vi "Read url 1.vi"(8 "error in (no error)":errorcluster, 11 "Firebase in":refnum<class "Firebase.lvclass">) -> (0 "error out":errorcluster, 2 "url":string, 3 "Firebase out":refnum<class "Firebase.lvclass">)   [LabVIEW 2019, in "Firebase.lvclass"]
uses:
  Firebase.lvclass
  Firebase.lvclass/Firebase.ctl
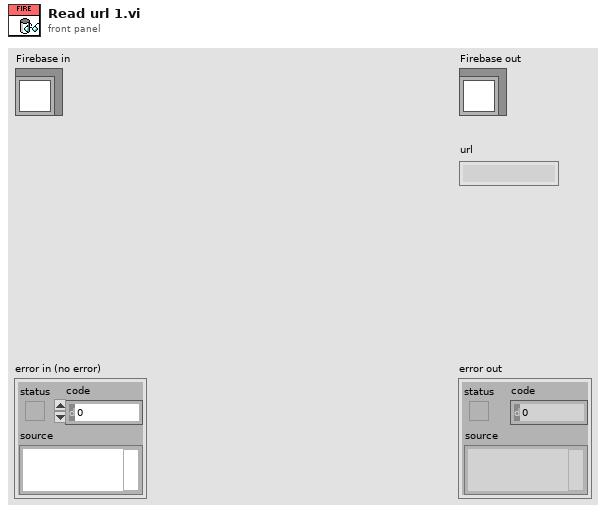
[diagram p1: front panel]
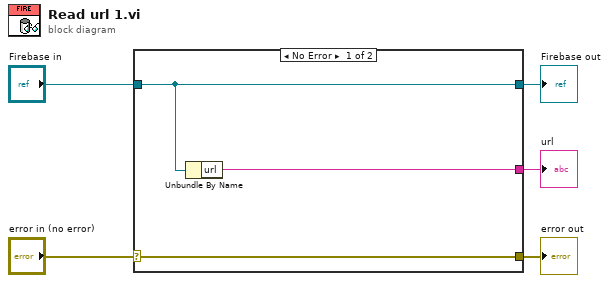
[diagram p0: block diagram]
diagram:
  n1 = case shown="No Error" "error in (no error)" {
    selector: "error in (no error)" -> [w8 w9]
    tunnel: [w8 w9] -> w4
    tunnel: [w7 w10] -> w2
    tunnel: "Firebase in" -> [w7 w10]
    tunnel: [w6 _] -> w1
    frame No Error {
      n2 = Unbundle By Name(w7) -> ("url"=w6:string)
    }
    frame Error {
    }
  }
  "error out" <- w4
  "Firebase out" <- w2
  "url" <- w1
